vi "ACT_SetpGradientFunction.vi"() -> ()   [LabVIEW 2022 SP3, in "MD420.lvclass"]
uses:
  MD420.lvclass
  MD420.lvclass/MD420.ctl
panel:
  out "gradient":dbl
  out "Gradient":dbl
  in  "Input":dbl
  in  "IAd":dbl
  in  "MD420.lvclass":refnum<class "MD420.lvclass">
  out "error out":errorcluster
  in  "error in":errorcluster
  in  "mode":enum16{"rapid", "by gradient"}(ring)
  out "Output":dbl
  in  "IC":bool
  in  "ULL":dbl
  in  "ILL":dbl
  in  "Igrd":dbl
  in  "I-":dbl
  in  "I+":dbl
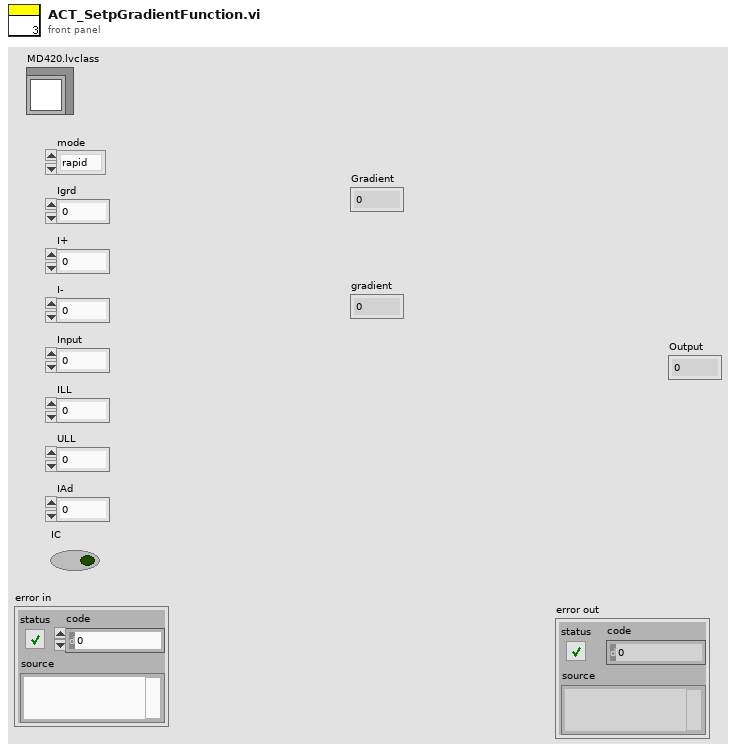
[diagram p1: front panel]
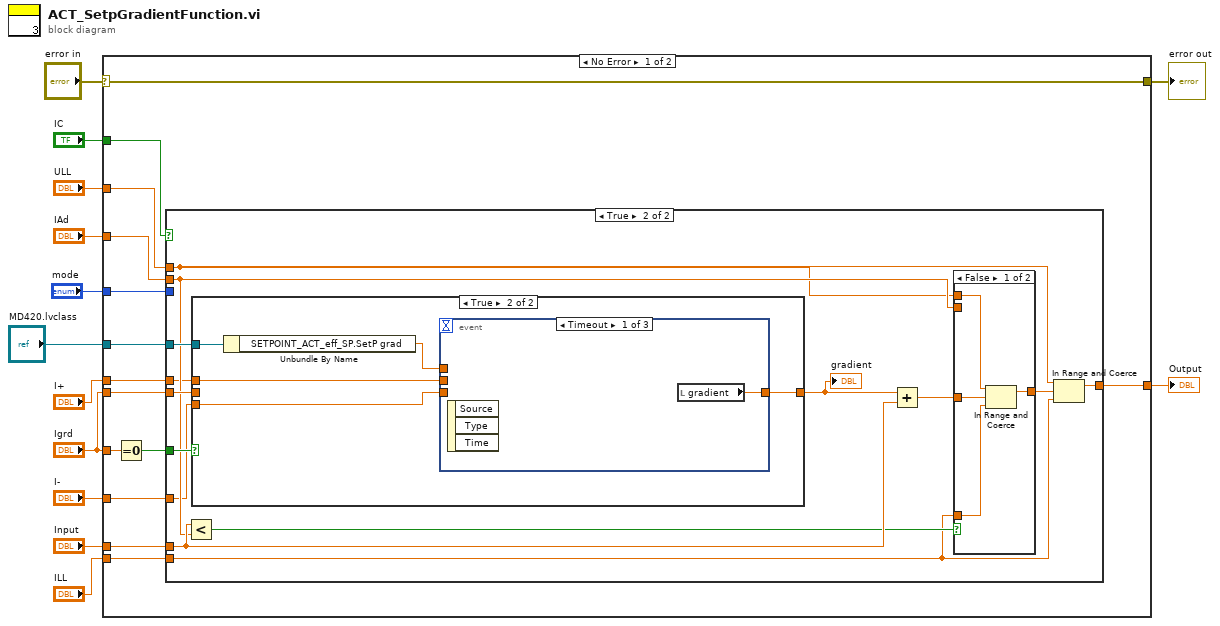
[diagram p0: block diagram]
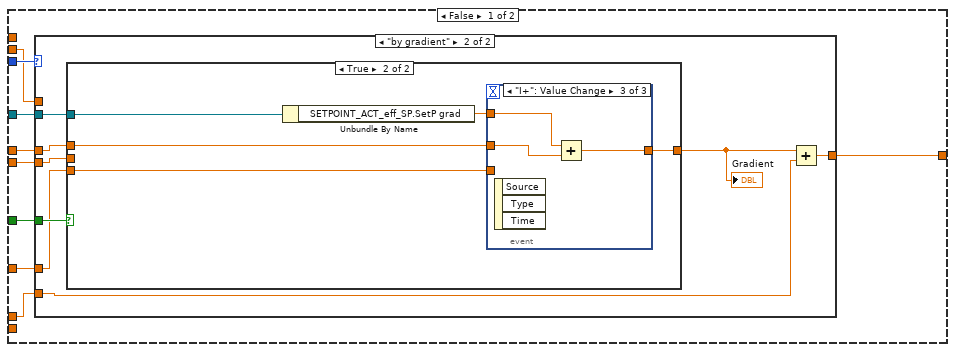
[diagram p2: hidden frame]
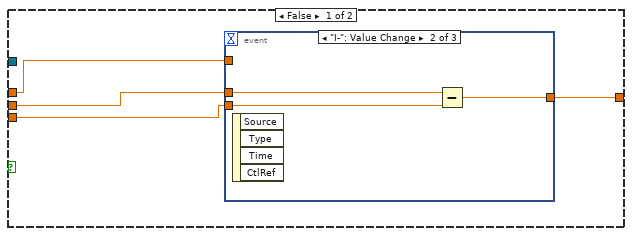
[diagram p4: hidden frame]
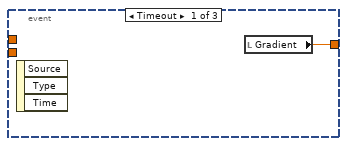
[diagram p5: hidden frame]
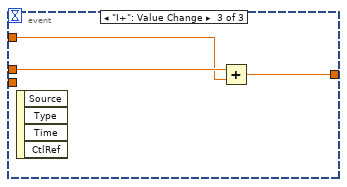
[diagram p6: hidden frame]
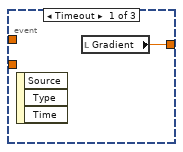
[diagram p7: hidden frame]
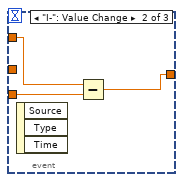
[diagram p8: hidden frame]
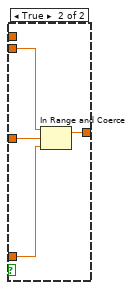
[diagram p9: hidden frame]
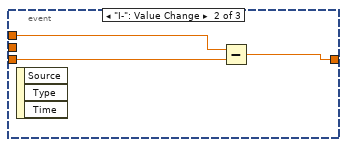
[diagram p11: hidden frame]
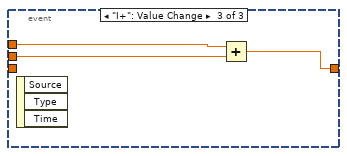
[diagram p12: hidden frame]
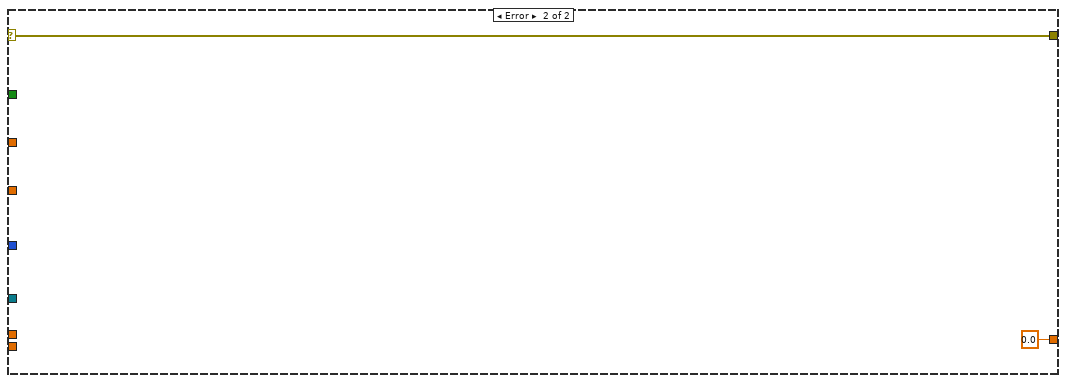
[diagram p13: hidden frame]
diagram:
  n1 = case shown="No Error" "error in" {
    selector: "error in" -> [w16 w104]
    tunnel: "Igrd" -> [w22 _]
    tunnel: "MD420.lvclass" -> [w27 _]
    tunnel: "mode" -> [w26 _]
    tunnel: "IC" -> [w24 _]
    tunnel: "IAd" -> [w25 _]
    tunnel: [w21 0.0 ("IAd")] -> w8
    tunnel: "Input" -> [w20 _]
    tunnel: "Igrd" -> [w19 _]
    tunnel: "ILL" -> [w18 _]
    tunnel: "ULL" -> [w17 _]
    tunnel: [w16 w104] -> w3
    tunnel: "I+" -> [w15 _]
    tunnel: "I-" -> [w14 _]
    frame No Error {
      n2 = Equal To 0?(x=w22) -> (x = 0?=w23:bool)
      n3 = case shown="True" w24 {
        tunnel: w27 -> [w36 w82]
        tunnel: w26 -> [w35 _]
        tunnel: w25 -> [w34 w76]
        tunnel: w23 -> [w33 w81]
        tunnel: [w32 w69] -> w21
        tunnel: w20 -> [w31 w78]
        tunnel: w19 -> [w30 w79]
        tunnel: w18 -> [_ w70]
        tunnel: w17 -> [_ w71]
        tunnel: w15 -> [w29 w74]
        tunnel: w14 -> [w28 w73]
        frame False {
          n4 = case shown="\"by gradient\"" w35 {
            tunnel: w36 -> [_ w45]
            tunnel: w34 -> [w37 _]
            tunnel: w33 -> [_ w44]
            tunnel: [w37 w41] -> w32
            tunnel: w31 -> [_ w43]
            tunnel: w30 -> [_ w42]
            tunnel: w29 -> [_ w40]
            tunnel: w28 -> [_ w39]
            frame "rapid", Default {
            }
            frame "by gradient" {
              n5 = case shown="True" w44 {
                tunnel: w45 -> [_ w61]
                tunnel: [w47 w57] -> w38
                tunnel: w42 -> [w48 _]
                tunnel: w40 -> [w49 w59]
                tunnel: w39 -> [w46 w58]
                frame False {
                  n6 = event shown="[1] \"I-\": Value Change" {
                    selector: _ -> [_ _ _]
                    dyn-events: _ -> [_ _ _]
                    timeout: _ -> [_ _ _]
                    tunnel: w49 -> [_ _ w55]
                    tunnel: w48 -> [_ w52 w56]
                    tunnel: [w50 w51 w54] -> w47
                    tunnel: w46 -> [_ w53 _]
                    event Timeout {
                      n7 = event-data() -> ()  [unwired: 1 in, 3 out]
                      n8 = local read "Gradient"() -> (w50:dbl)
                    }
                    event "I-": Value Change {
                      n9 = event-data() -> ()  [unwired: 1 in, 4 out]
                      n10 = Subtract(x=w52, y=w53) -> (x-y=w51:dbl)
                    }
                    event "I+": Value Change {
                      n11 = event-data() -> ()  [unwired: 1 in, 4 out]
                      n12 = Add(x=w56, y=w55) -> (x+y=w54:dbl)
                    }
                  }
                }
                frame True {
                  n13 = Unbundle By Name(w61) -> ("SETPOINT_ACT_eff_SP.SetP grad"=w60:dbl)
                  n14 = event shown="[2] \"I+\": Value Change" {
                    selector: _ -> [_ _ _]
                    dyn-events: _ -> [_ _ _]
                    timeout: _ -> [_ _ _]
                    tunnel: w60 -> [_ w65 w67]
                    tunnel: w59 -> [_ _ w66]
                    tunnel: w58 -> [_ w64 _]
                    tunnel: [w62 w63 w68] -> w57
                    event Timeout {
                      n15 = event-data() -> ()  [unwired: 1 in, 3 out]
                      n16 = local read "Gradient"() -> (w62:dbl)
                    }
                    event "I-": Value Change {
                      n17 = event-data() -> ()  [unwired: 1 in, 3 out]
                      n18 = Subtract(x=w65, y=w64) -> (x-y=w63:dbl)
                    }
                    event "I+": Value Change {
                      n19 = event-data() -> ()  [unwired: 1 in, 3 out]
                      n20 = Add(x=w67, y=w66) -> (x+y=w68:dbl)
                    }
                  }
                }
              }
              "Gradient" <- w38
              n21 = Add(x=w38, y=w43) -> (x+y=w41:dbl)
            }
          }
        }
        frame True {
          n22 = Less?(x=w78, y=w76) -> (x < y?=w77:bool)
          n23 = case shown="True" w81 {
            tunnel: w82 -> [_ w96]
            tunnel: [w91 w93] -> w80
            tunnel: w79 -> [w91 _]
            tunnel: w74 -> [_ w94]
            tunnel: w73 -> [_ w92]
            frame False {
            }
            frame True {
              n24 = Unbundle By Name(w96) -> ("SETPOINT_ACT_eff_SP.SetP grad"=w95:dbl)
              n25 = event shown="[0] Timeout" {
                selector: _ -> [_ _ _]
                dyn-events: _ -> [_ _ _]
                timeout: _ -> [_ _ _]
                tunnel: w95 -> [_ w100 w103]
                tunnel: w94 -> [_ _ w102]
                tunnel: [w97 w98 w101] -> w93
                tunnel: w92 -> [_ w99 _]
                event Timeout {
                  n26 = event-data() -> ()  [unwired: 1 in, 3 out]
                  n27 = local read "gradient"() -> (w97:dbl)
                }
                event "I-": Value Change {
                  n28 = event-data() -> ()  [unwired: 1 in, 3 out]
                  n29 = Subtract(x=w100, y=w99) -> (x-y=w98:dbl)
                }
                event "I+": Value Change {
                  n30 = event-data() -> ()  [unwired: 1 in, 3 out]
                  n31 = Add(x=w103, y=w102) -> (x+y=w101:dbl)
                }
              }
            }
          }
          "gradient" <- w80
          n32 = Add(x=w80, y=w78) -> (x+y=w75:dbl)
          n33 = case shown="False" w77 {
            tunnel: w76 -> [_ w90]
            tunnel: w70 -> [w86 w89]
            tunnel: w75 -> [w84 w88]
            tunnel: w71 -> [w85 _]
            tunnel: [w83 w87] -> w72
            frame False {
              n34 = In Range and Coerce(upper limit=w85, x=w84, lower limit=w86) -> (coerced(x)=w83:dbl)  [unwired: 1 out]
            }
            frame True {
              n35 = In Range and Coerce(upper limit=w90, x=w88, lower limit=w89) -> (coerced(x)=w87:dbl)  [unwired: 1 out]
            }
          }
          n36 = In Range and Coerce(upper limit=w71, x=w72, lower limit=w70) -> (coerced(x)=w69:dbl)  [unwired: 1 out]
        }
      }
    }
    frame Error {
    }
  }
  "Output" <- w8
  "error out" <- w3
